vi "SetExitEvent.vi"(8 "error in (no error)":errorcluster, 10 "ExitEvent":refnum<user-event>, 11 "ClassByRef in":refnum<class "ClassByRef.lvclass">) -> (0 "error out":errorcluster, 3 "ClassByRef out":refnum<class "ClassByRef.lvclass">)   [LabVIEW 2021, in "ClassUtilities.lvlib" / "ClassByRef.lvclass"]
uses:
  ClassByRef.lvclass
  ClassByRef.lvclass/ClassByRef.ctl
  bebabc09-0ae7-43ee-9c47-cce95fb00d63.vi
  GetRef.vi
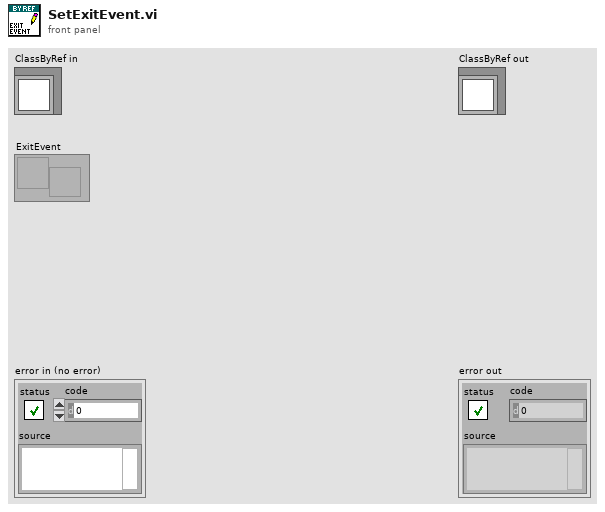
[diagram p1: front panel]
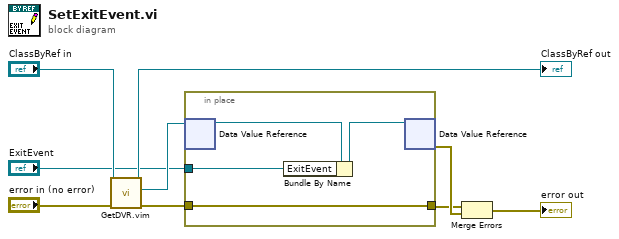
[diagram p0: block diagram]
diagram:
  n1 = call "GetDVR.vim"("error in (no error)"="error in (no error)", "ByRefClass in"="ClassByRef in") -> ("error out"=w2:errorcluster, "DVR"=w4:refnum<data-value>, "ByRefClass out"=→"ClassByRef out":refnum<class "ClassByRef.lvclass">)  [unwired: 7 in]
  n2 = in-place {
    in-place-border: w2 -> [w13]
    in-place-border: [w13] -> w7
    in-place-border: "ExitEvent" -> [w10]
    n3 = in-place-dvr #1(w4) -> (w11:refnum<class "ClassByRef.lvclass">)  [unwired: 1 out]
    n4 = Bundle By Name(cluster=w11, "ExitEvent"=w10) -> (w12:refnum<class "ClassByRef.lvclass">)
    n5 = in-place-dvr #1(w12) -> (w8:errorcluster)  [unwired: 1 out]
  }
  n6 = Merge Errors(w7, w8) -> (→"error out":errorcluster)
